vi "Zero Select K Rows.vi"(7 "Reobserved Array":bool[](array[boolean]), 10 "K In":T1) -> (2 "K Out":T1)   [LabVIEW 2009]
uses:
  <vilib>/Analysis/Matrix/Datatypes/RealMatrix.ctl
  <vilib>/Analysis/Matrix/NI_Matrix.lvlib
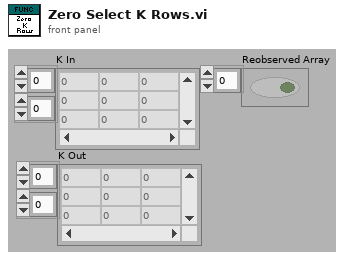
[diagram p1: front panel]
types:
  T1 = typedef "NI_Matrix.lvlib/RealMatrix.ctl" = dbl[][]
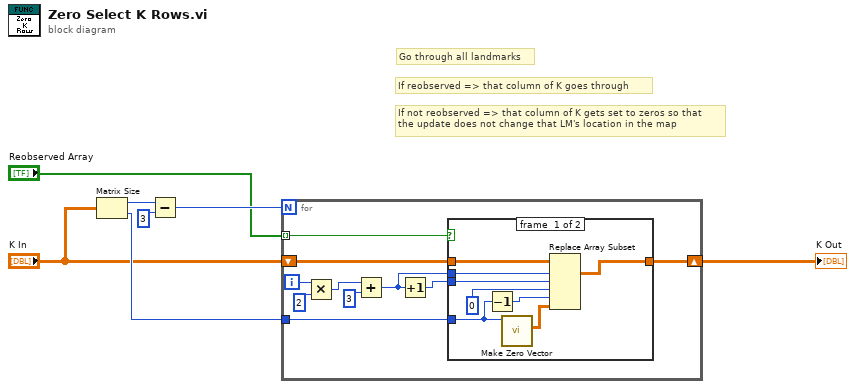
[diagram p0: block diagram]
diagram:
  # "If not reobserved => that column of K gets set to zeros so that\nthe update does not change that LM's location in the map"
  # "If reobserved => that column of K goes through"
  # "Go through all landmarks"
  n1 = Matrix Size(0:"K In") -> (1:w6:i32, 2:w4:i32)
  n2 = Subtract(x=w6, y=3) -> (x-y=w7:i32)
  n3 = for {
    N: w7 -> [_]
    tunnel: "Reobserved Array" -> [w13] mode=indexing
    shift-right: [w17] -> w3
    shift-left: "K In" -> [w16]
    tunnel: w4 -> [w14]
    i -> [w9]
    n4 = Multiply(x=w9, y=2) -> (x*y=w8:i32)
    n5 = Add(x=w8, y=3) -> (x+y=w11:i32)
    n6 = Increment(x=w11) -> (x+1=w15:i32)
    n7 = case shown="False" w13 {
      tunnel: [w24 w26] -> w17
      tunnel: w16 -> [w25 w26]
      tunnel: w11 -> [w23 _]
      tunnel: w15 -> [w22 _]
      tunnel: w14 -> [w20 _]
      frame #0 {
        n8 = Decrement(x=w20) -> (x-1=w19:i32)
        n9 = call "Make Zero Vector.vi"("Columns"=w20) -> ("Zero Vector"=w18:T1)  [unwired: 10 in]
        n10 = Replace Array Subset(array=w25, new element=w18, index (dim 0)=w23, index (dim 1)=w22, index (dim 2)=0 ("column 1"), index (dim 3)=w19) -> (w24:T1)
      }
      frame #1 {
      }
    }
  }
  "K Out" <- w3
